vi "main_with_data.vi"() -> ()   [LabVIEW 2024]
panel:
  out "Numeric":dbl
  in  "Knob":dbl(knob) scale=0.0..10.0
  in  "stop":bool
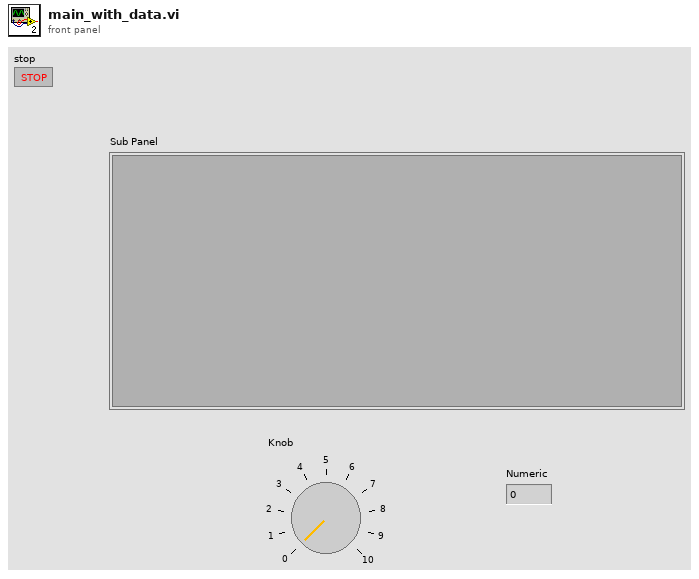
[diagram p1: front panel]
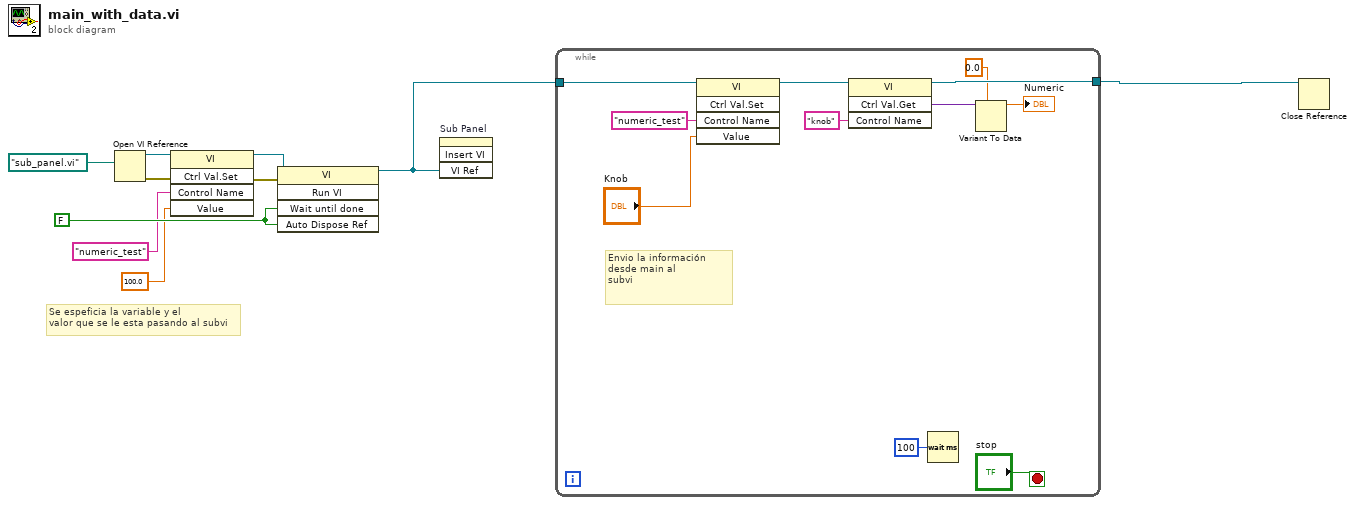
[diagram p0: block diagram]
diagram:
  w6 = FALSE ("Wait Until Done")
  # "Se espeficia la variable y el \nvalor que se le esta pasando al subvi"
  n1 = Open VI Reference(vi path=path "sub_panel.vi") -> (vi reference=w8:refnum<vi>, error out=w7:errorcluster)  [unwired: 5 in]
  n2 = invoke class="VI" method="Ctrl Val.Set"(reference=w8, "Control Name"="numeric_test", "Value"=100.0) -> (reference out=w3:refnum<vi>)  [unwired: 2 in, 4 out]
  n3 = invoke class="VI" method="Run VI"(reference=w3, error in=w7, "Wait until done"=w6, "Auto Dispose Ref"=w6) -> (reference out=w5:refnum<vi>)  [unwired: 1 in, 4 out]
  n4 = invoke on="Sub Panel" class="SubPnl" method="Insert VI"("VI Ref"=w5) -> ()  [unwired: 3 in, 4 out]
  n5 = while {
    tunnel: w5 -> [w19]
    tunnel: [w14] -> w4
    stop <- "stop" stop-if-true
    # "Envio la información desde main al \nsubvi"
    n6 = invoke class="VI" method="Ctrl Val.Set"(reference=w19, "Control Name"="numeric_test", "Value"="Knob") -> (reference out=w17:refnum<vi>)  [unwired: 2 in, 4 out]
    n7 = invoke class="VI" method="Ctrl Val.Get"(reference=w17, "Control Name"="knob") -> (reference out=w14:refnum<vi>, "Get Control Value Variant"=w12:variant)  [unwired: 2 in, 2 out]
    n8 = Wait (ms)(milliseconds to wait=u32 100) -> ()  [unwired: 1 out]
    n9 = Variant To Data(type=0.0, Variant=w12) -> (data=→"Numeric":dbl)  [unwired: 1 in, 1 out]
  }
  n10 = Close Reference(reference=w4) -> ()  [unwired: 1 in, 1 out]
